vi "Times Global.vi"() -> ()   [LabVIEW 2018]
panel:
  out "Cargo Delta Time Graph":u32(graph)
  in  "On/Off Hab Climber PT 3":bool
  in  "Hatch Panel Loop Time":dbl=40.0
  in  "On/Off Hab Climber PT 2":bool
  in  "Lift Loop Time":dbl=20.0
  in  "On/Off Driver Controls PT 2":bool
  in  "Manipulator Controls Loop Time":dbl=20.0
  in  "On/Off Hab Climber PT":bool
  in  "On/Off Sensors PT":bool
  in  "On/Off Swerve Drive PT":bool
  in  "On/Off Driver Controls PT":bool
  in  "Hab Climber Loop Time":dbl=50.0
  in  "Driver Controls Loop Time":dbl=20.0
  in  "Cargo Intake Loop Time":dbl=40.0
  in  "Swerve Drive Loop Time":dbl=20.0
  # "Loop Times"
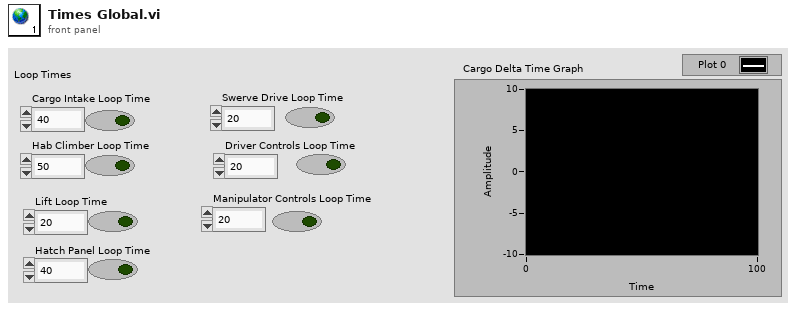
[diagram p1: front panel]
diagram:
